vi "Read Allow Zeroing.vi"(8 "error in (no error)":errorcluster, 11 "Power Meter Base in":refnum<class "Power Meter Base.lvclass">) -> (0 "error out":errorcluster, 2 "Allow Zeroing":bool, 3 "Power Meter Base out":refnum<class "Power Meter Base.lvclass">)   [LabVIEW 2023, in "RFFixtureCharact.Instruments.lvlib" / "Power Meter Base.lvclass"]
uses:
  Power Meter Base.lvclass
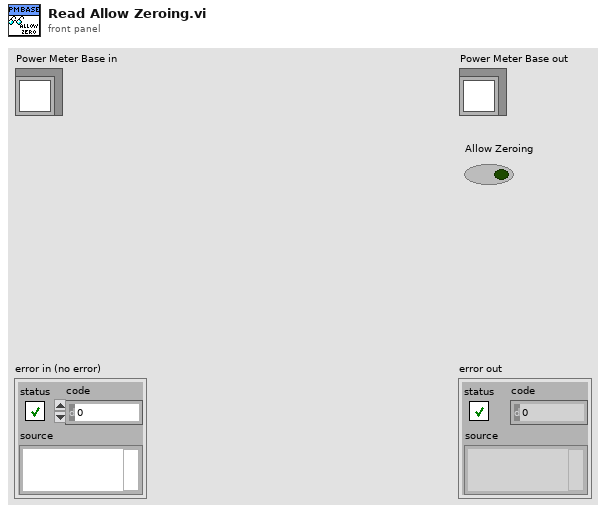
[diagram p1: front panel]
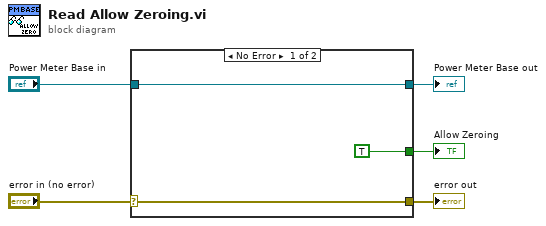
[diagram p0: block diagram]
diagram:
  n1 = case shown="No Error" "error in (no error)" {
    selector: "error in (no error)" -> [w8 w9]
    tunnel: [w8 w9] -> w4
    tunnel: [w7 w10] -> w2
    tunnel: "Power Meter Base in" -> [w7 w10]
    tunnel: [TRUE ("Allow Zeroing") _] -> w1
    frame No Error {
    }
    frame Error {
    }
  }
  "error out" <- w4
  "Power Meter Base out" <- w2
  "Allow Zeroing" <- w1
